vi "Fitts.vi"(11 "ID":dbl) -> (1 "W":dbl, 2 "D":dbl)   [LabVIEW 2010]
panel:
  out "lD":dbl
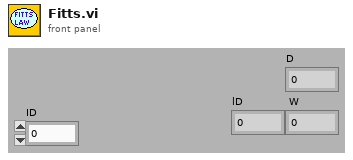
[diagram p1: front panel]
types:
  T1 = typedef "LVAllMonitorsDisplayTypeDef.ctl" = cluster{"Bounds":cluster{"Left":i16, "Top":i16, "Right":i16, "Bottom":i16}, "Depth":i16}[]
  T2 = cluster{"Bounds":cluster{"Left":i16, "Top":i16, "Right":i16, "Bottom":i16}, "Depth":i16}
  T3 = cluster{"Left":i16, "Top":i16, "Right":i16, "Bottom":i16}
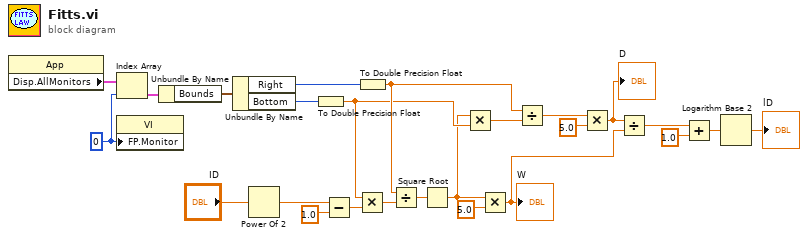
[diagram p0: block diagram]
diagram:
  w25 = u16 0 ("Front Panel Window:Monitor")
  n1 = property class="App"() -> ("Disp.AllMonitors"=w24:T1)  [unwired: 2 in, 2 out]
  n2 = Index Array(array=w24, index=w25) -> (element=w23:T2)
  n3 = property class="VI"("FP.Monitor"=w25) -> ()  [unwired: 2 in, 2 out]
  n4 = Unbundle By Name(w23) -> ("Bounds"=w22:T3)
  n5 = Unbundle By Name(w22) -> ("Right"=w9:i16, "Bottom"=w8:i16)
  n6 = Power Of 2(x="ID") -> (2^x=w19:dbl)
  n7 = To Double Precision Float(number=w8) -> (double precision float=w15:dbl)
  n8 = Subtract(x=w19, y=1.0) -> (x-y=w17:dbl)
  n9 = Multiply(x=w15, y=w17) -> (x*y=w21:dbl)
  n10 = To Double Precision Float(number=w9) -> (double precision float=w16:dbl)
  n11 = Divide(x=w16, y=w21) -> (x/y=w20:dbl)
  n12 = Square Root(x=w20) -> (sqrt(x)=w4:dbl)
  n13 = Multiply(x=w4, y=w15) -> (x*y=w14:dbl)
  n14 = Multiply(x=w4, y=5.0) -> (x*y=w3:dbl)
  "W" <- w3
  n15 = Divide(x=w16, y=w14) -> (x/y=w7:dbl)
  n16 = Multiply(x=w7, y=5.0) -> (x*y=w2:dbl)
  "D" <- w2
  n17 = Divide(x=w2, y=w3) -> (x/y=w13:dbl)
  n18 = Add(x=w13, y=1.0) -> (x+y=w11:dbl)
  n19 = Logarithm Base 2(1:w11) -> (0:→"lD":dbl)
